vi "Dashboard Main.vi"() -> ()   [LabVIEW 2016]
uses:
  <vilib>/Utility/miscctls.llb/LVRowAndColumnTypeDef.ctl
  <vilib>/event_ctls.llb/eventvkey.ctl
  <vilib>/Rock Robotics/Network Tables/NT Read Numeric Array.vi
  <vilib>/Rock Robotics/Network Tables/NT Write Boolean.vi
  <vilib>/Rock Robotics/WPI/Dashboard/WPI_DashboardLogging Global.vi
panel:
  out "Background":bool
  in  "Camera Settings Right":T1={"Frame Rate"=30, "Compression"=30, "Size"=1, "DB Camera Config"=FALSE} {"Frame Rate" scale=1.0..30.0; "Compression" scale=100.0..-1.0; "Size" items=["640x480", "320x240", "160x120"]}
  in  "Camera Name Right":string(combo)="No Camera Selection"
  out "Camera Info":cluster{"Mbps LED":bool, "Mbps":dbl, "fps":dbl} {"fps" format="%#.1g"; "Mbps" format="%#.1g"}
  in  "Camera Settings":T1={"Frame Rate"=30, "Compression"=30, "Size"=1, "DB Camera Config"=FALSE} {"Frame Rate" scale=1.0..30.0; "Compression" scale=100.0..-1.0; "Size" items=["640x480", "320x240", "160x120"]}
  in  "TCP":refnum<k5>
  in  "Rec Mode":enum32{"Stop", "Record", "Playback"}(radio)
  out "Robot IP":string
  out "Image Message":string="Timeout in Camera Communications"
  in  "Dashboard Tab":T2(tab)
  in  "Smooth":i32(knob) scale=1.0..4.0
  in  "GoFast":bool
  in  "Select Auto":string(combo)="Select Autonomous ..."
  out "NT Connection":bool
  out "MotorChart R":cluster{"Numeric":dbl, "Numeric":dbl}(graph)
  out "MotorChart L":cluster{"Numeric":dbl, "Numeric":dbl}(graph)
  out "MotorSliders R":cluster{"MotorSlide1":dbl, "MotorSlide2":dbl} {"MotorSlide2" scale=-1.0..1.0 scale format="%#_2e"; "MotorSlide1" scale=-1.0..1.0 scale format="%#_2e"}
  out "MotorSliders L":cluster{"MotorSlide1":dbl, "MotorSlide2":dbl} {"MotorSlide2" scale=-1.0..1.0 scale format="%#_2e"; "MotorSlide1" scale=-1.0..1.0 scale format="%#_2e"}
  out "Gyro":dbl(knob) scale=0.0..360.0
  out "JS1 Z":dbl(slide) scale=-1.0..1.0 scale format="%#_2e"
  out "JS1 Graph":cluster{"X":dbl, "Y":dbl}[](graph)
  out "JS1 Buttons":T3
  out "JS2 Z":dbl(slide) scale=-1.0..1.0 scale format="%#_2e"
  out "JS2 Graph":cluster{"X":dbl, "Y":dbl}[](graph)
  out "JS2 Buttons":T3
  out "Mode":T4(ring)=enum."Auto Disabled"
  in  "Trim":dbl(slide)=0.5612244897959183 scale=0.0..1.0
  out "Sonar":dbl
  out "Camera Image Right":T5(plugin-control)
  in  "Calculate Angle":bool
  in  "Angle to turn":dbl=30.0
  out "Angle":dbl
  in  "Distance from\n lift to corner":dbl
  in  "Distance from \nthe lift to the wall":dbl
  in  "DB/String 4":string
  in  "DB/String 3":string
  in  "DB/String 2":string
  in  "DB/String 1":string
  in  "DB/String 0":string
  in  "DB/Slider 0":dbl(slide)=0.65 caption="Turning Speed" scale=0.0..1.0
  in  "DB/Slider 1":dbl(slide)=11.0 caption="Distance we stop\nfrom lift (in inches)" scale=0.0..30.0
  in  "DB/Slider 2":dbl(slide)=11.111111111111112 caption="Autonomous Stop" scale=0.0..50.0
  in  "DB/Slider 3":dbl(slide)=0.6565656565656566 caption="Autonomous Trim" scale=0.0..1.0
  out "DB/LED 3":bool
  out "DB/LED 2":bool
  out "DB/LED 1":bool
  out "DB/LED 0":bool
  in  "DB/Button 3":bool
  in  "DB/Button 2":bool
  in  "DB/Button 1":bool
  in  "DB/Button 0":bool caption="New Name"
  in  "Scaling factor (V/in)":dbl=0.0098
  out "distance":dbl(slide)=125.0 scale=0.0..250.0 scale format="%3d"
  out "Z Acceleration":dbl
  out "Y Acceleration":dbl
  out "X Acceleration":dbl
  in  "Test Slider":dbl(slide) scale=0.0..100.0 scale format="%#_3g"
  in  "On/Off":bool caption="Solenoid"
  in  "Test Name":u16(ring) items=["Select the test to run..."]
  in  "Test Tree":string(tree)
  in  "Motor":cluster{"Value":dbl, "Enable":bool} {"Value" scale=-1.0..1.0 scale format="%#_3g"}
  out "Progress":T6 {"Test Progress" scale=0.0..100.0}
  in  "Rev/Fwd":cluster{"Forward":bool, "Reverse":bool}
  in  "Test Ring":u16(ring) items=["Monochrome", "Color"]
  out "Cmd Status":string
  in  "Execute Command":bool
  in  "Command Params":string[][](table)
  in  "Command Selection":i32(listbox)
  in  "CheckList":i32(listbox)
  out "Tree":string(tree)
  out "Camera Image":T5(plugin-control)
  in  "Camera Name":string(combo)="No Camera Selection"
  # "HW"
  # "HW"
  # "Joysticks"
  # "Drive Motors"
  # "Front"
  # "Right"
  # "Left"
  # "Back"
  # "This tab is a great place for autonomous settings and robot-specific values.\nPlace controls and indicators inside this tab and match name to\nDashboard Variables on robot. You can also delete this comment."
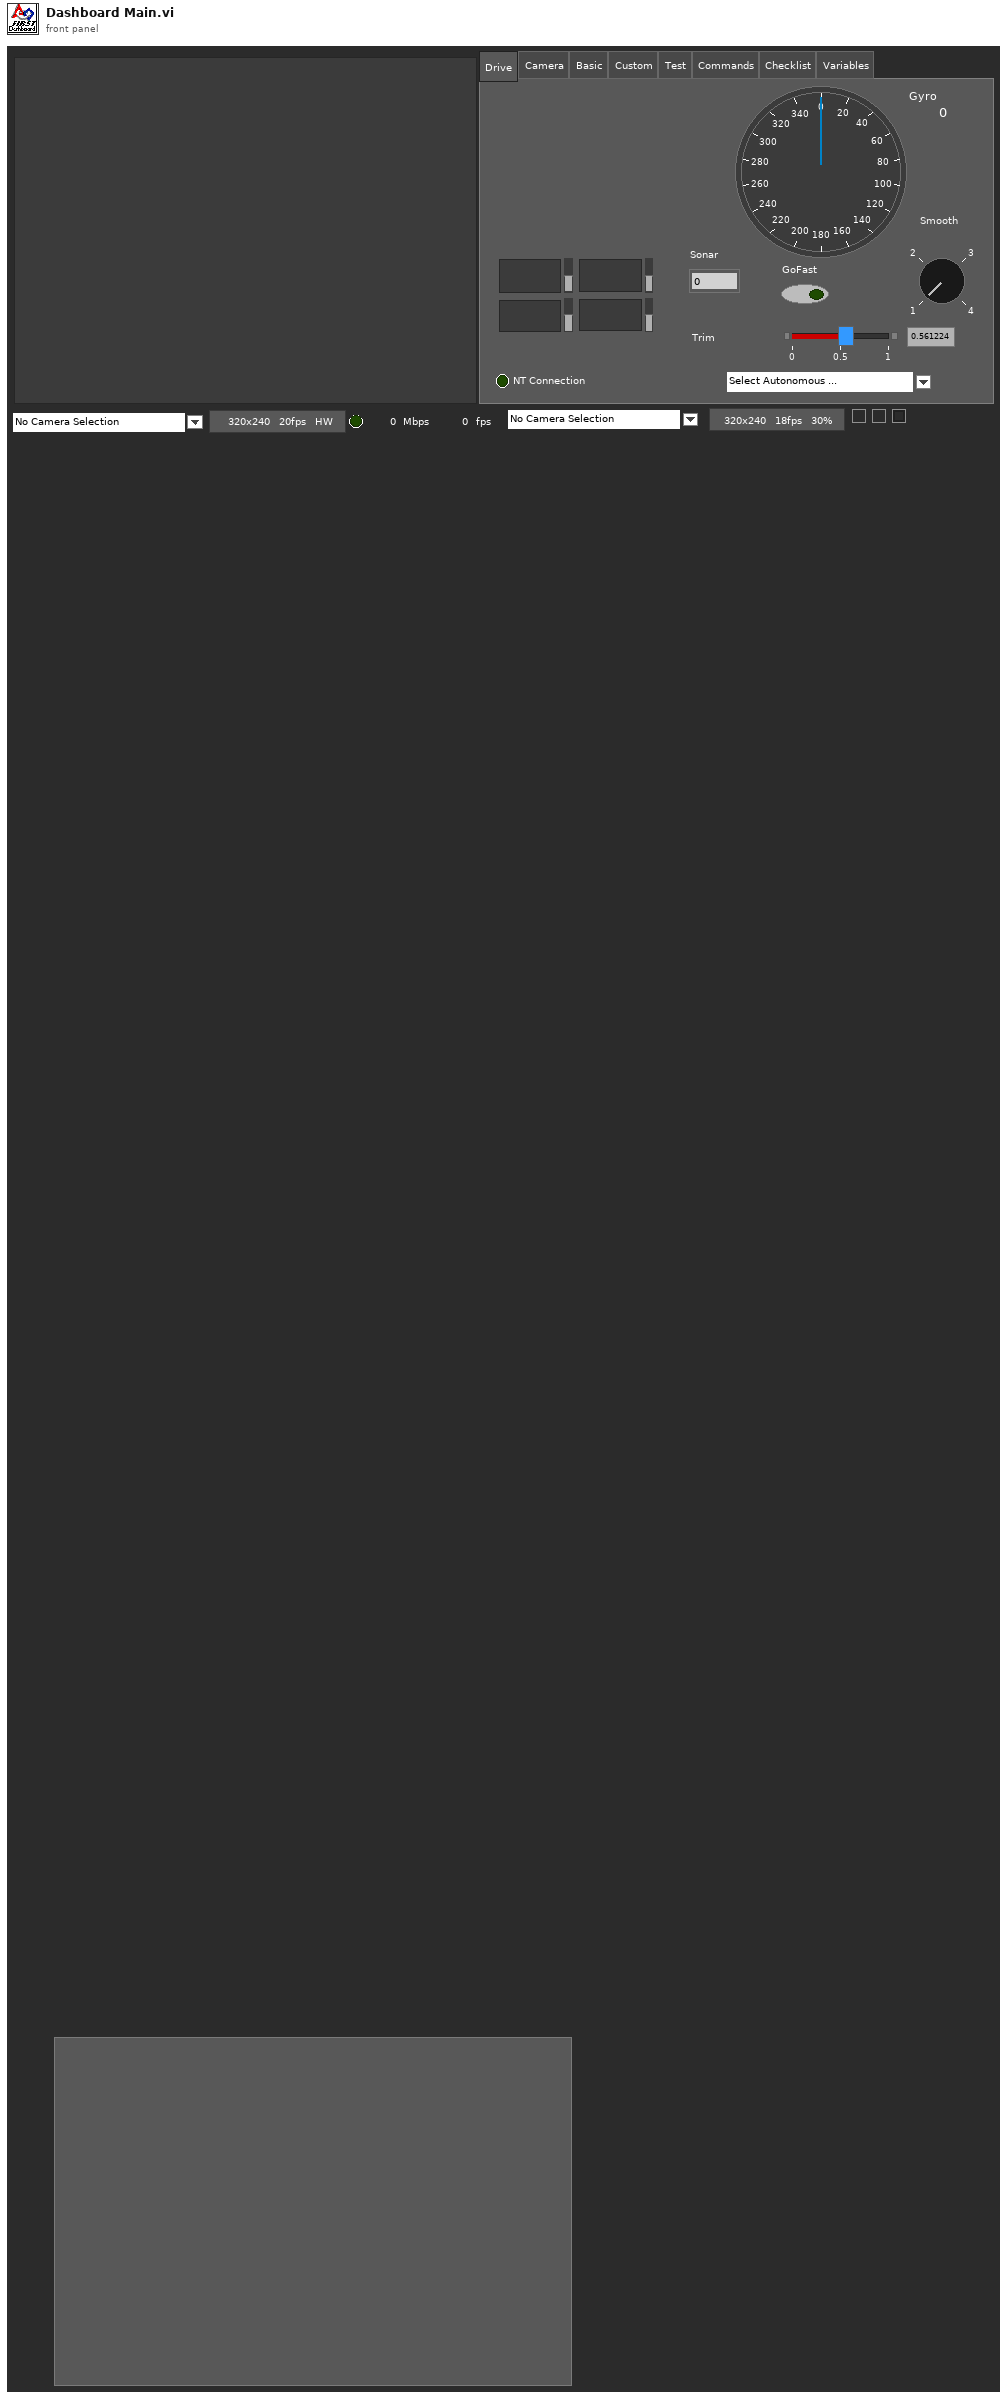
[diagram p1: front panel]
types:
  T1 = cluster{"Frame Rate":i32, "Compression":i32, "Size":u16, "DB Camera Config":bool}
  T2 = enum32{"Drive", "Camera", "Basic", "Custom", "Test", "Commands", "Checklist", "Variables"}
  T3 = cluster{bool, bool, bool, bool, bool, bool, bool, bool, bool, bool, bool, bool}
  T4 = enum8{"Tele-Op Disabled", "Tele-Op Enabled", "Auto Disabled", "Auto Enabled", "Test Disabled", "Test Enabled", "Disconnected", "No Code", "E-Stop"}
  T5 = typedef "IMAQ Image.ctl" = refnum<image>
  T6 = cluster{"Test Progress":u8, "Test Progress Text":string}
  T7 = typedef "Image Type" = u32
  T8 = cluster{"IDs":cluster{"RPC field ID":u16, "Unique ID":u16}, "String":string}
  T9 = enum32{"Drive", "Basic", "Custom", "Test", "Checklist", "Variables"}
  T10 = cluster{"Error Strings":string, "Disable Counts":cluster{u16, u16}, "Rail Faults":cluster{u16, u16, u16}, "Robot IP":string, "DB Mode":u8, "Event Info":cluster{"Name":string, "Type":u8, "Number":u16, "Replay":u8}}
  T11 = cluster{"Storage":cluster{"Disk Free":u64, "RAM Block":u32, "RAM free":u32}, "CPU Utilization":cluster{"CPU % ISR":sgl, "CPU % Time Crit":sgl, "CPU % Timed Str":sgl, "CPU % High":sgl, "CPU % Above":sgl, "CPU % Normal":sgl, "CPU % Low":sgl}, "CAN":cluster{"% Bus Utilization":sgl, "Bus Off Cnt":u32, "TX_FIFO Full Cnt":u32, "Receive Error Cnt":u8, "Transmit Error Cnt":u8}, "HID":cluster{"HID Outputs":u32, "Rumble Low":u16, "Rumble High":u16}[]}
  T12 = cluster{"Status bits":cluster{"Test Mode":bool, "Autonomous":bool, "Enabled":bool, "Code Start":bool, "Brownout":bool, "Reserved 2":bool, "Reserved 3":bool, "E-Stop":bool}, "Code Trace":cluster{"Disabled":bool, "TeleOp":bool, "Auto":bool, "Test":bool}, "Controller Type":enum16{"unknown", "cRIO", "roboRio"}, "Code?":enum16{"unknown", "noCode", "code"}, "Battery V":dbl}
  T13 = cluster{"Control Bits":cluster{"TestMode":bool, "Autonomous":bool, "Enabled":bool, "FMS Present":bool, bool, bool, bool, "E-Stop":bool}, "Team Station ":u8, "Countdown":sgl, "Joystick Values":cluster{"Axes":dbl[], "Buttons":bool[], "POVs":i16[]}[]}
  T14 = cluster{"Axes":dbl[], "Buttons":bool[], "POVs":i16[]}[]
  T15 = cluster{"Axes":dbl[], "Buttons":bool[], "POVs":i16[]}
  T16 = cluster{"Buttons[0]":bool, "Buttons[1]":bool, "Buttons[2]":bool, "Buttons[3]":bool, "Buttons[4]":bool, "Buttons[5]":bool, "Buttons[6]":bool, "Buttons[7]":bool, "Buttons[8]":bool, "Buttons[9]":bool, "Buttons[10]":bool, "Buttons[11]":bool}
  T17 = cluster{"Camera Image":refnum<vi>, "Dashboard Tab":refnum<vi>, "Background":refnum<vi>, "Rec Mode":refnum<vi>, "Test Slider":refnum<vi>, "On/Off ":refnum<vi>, "Test Ring":refnum<vi>, "Rev/Fwd":refnum<vi>, "Test Name":refnum<vi>, "Motor":refnum<vi>, "Progress":refnum<vi>, "CheckList":refnum<vi>, "Tree":refnum<vi>, "Test Tree":refnum<vi>, "Command Params":refnum<vi>, "Command Selection":refnum<vi>, "Execute Command":refnum<vi>, "Cmd Status":refnum<vi>, "Camera Settings":refnum<vi>, "Camera Name":refnum<vi>, "Camera Info":refnum<vi>, "Camera Settings Right":refnum<vi>, "Camera Name Right":refnum<vi>, "Camera Image Right":refnum<vi>}
  T18 = cluster{"Operation":enum16{"Update", "Clear"}, "Color Box":u32}[]
  T19 = typedef "eventvkey.ctl" = enum16{"ASCII", "Enter", "Return", "Shift", "Ctrl", "Alt", "Cmd", "Opt", "Caps", "NumLock", "Clear", "Break", "Up", "Down", "Left", "Right", "Insert", "Delete", "Home", "End", "PageUp", "PageDown", "Escape", "Help", "Pause", "ScrollLock", "F1", "F2", "F3", "F4", "F5", "F6", "F7", "F8", "F9", "F10", "F11", "F12", "F13", "F14", "F15", "F16", "F17", "F18", "F19", "F20", "F21", "F22", "F23", "F24", "Play", "VolumeUp", "VolumeDown", "Mute", "Two Byte Char"}
  T20 = cluster{"Image Size":bool, "Image Type":bool, "Pixel Value":bool, "ROI Information":bool, "Zoom Factor":bool}
  T21 = cluster{"Operation":enum16{"Update", "Clear"}, "Color Box":u32}
  T22 = typedef "LVRowAndColumnTypeDef.ctl" = cluster{"Row":i32, "Column":i32}
  T23 = cluster{"Shift":bool, "Ctrl":bool, "Alt":bool, "Cmd":bool, "Opt":bool}
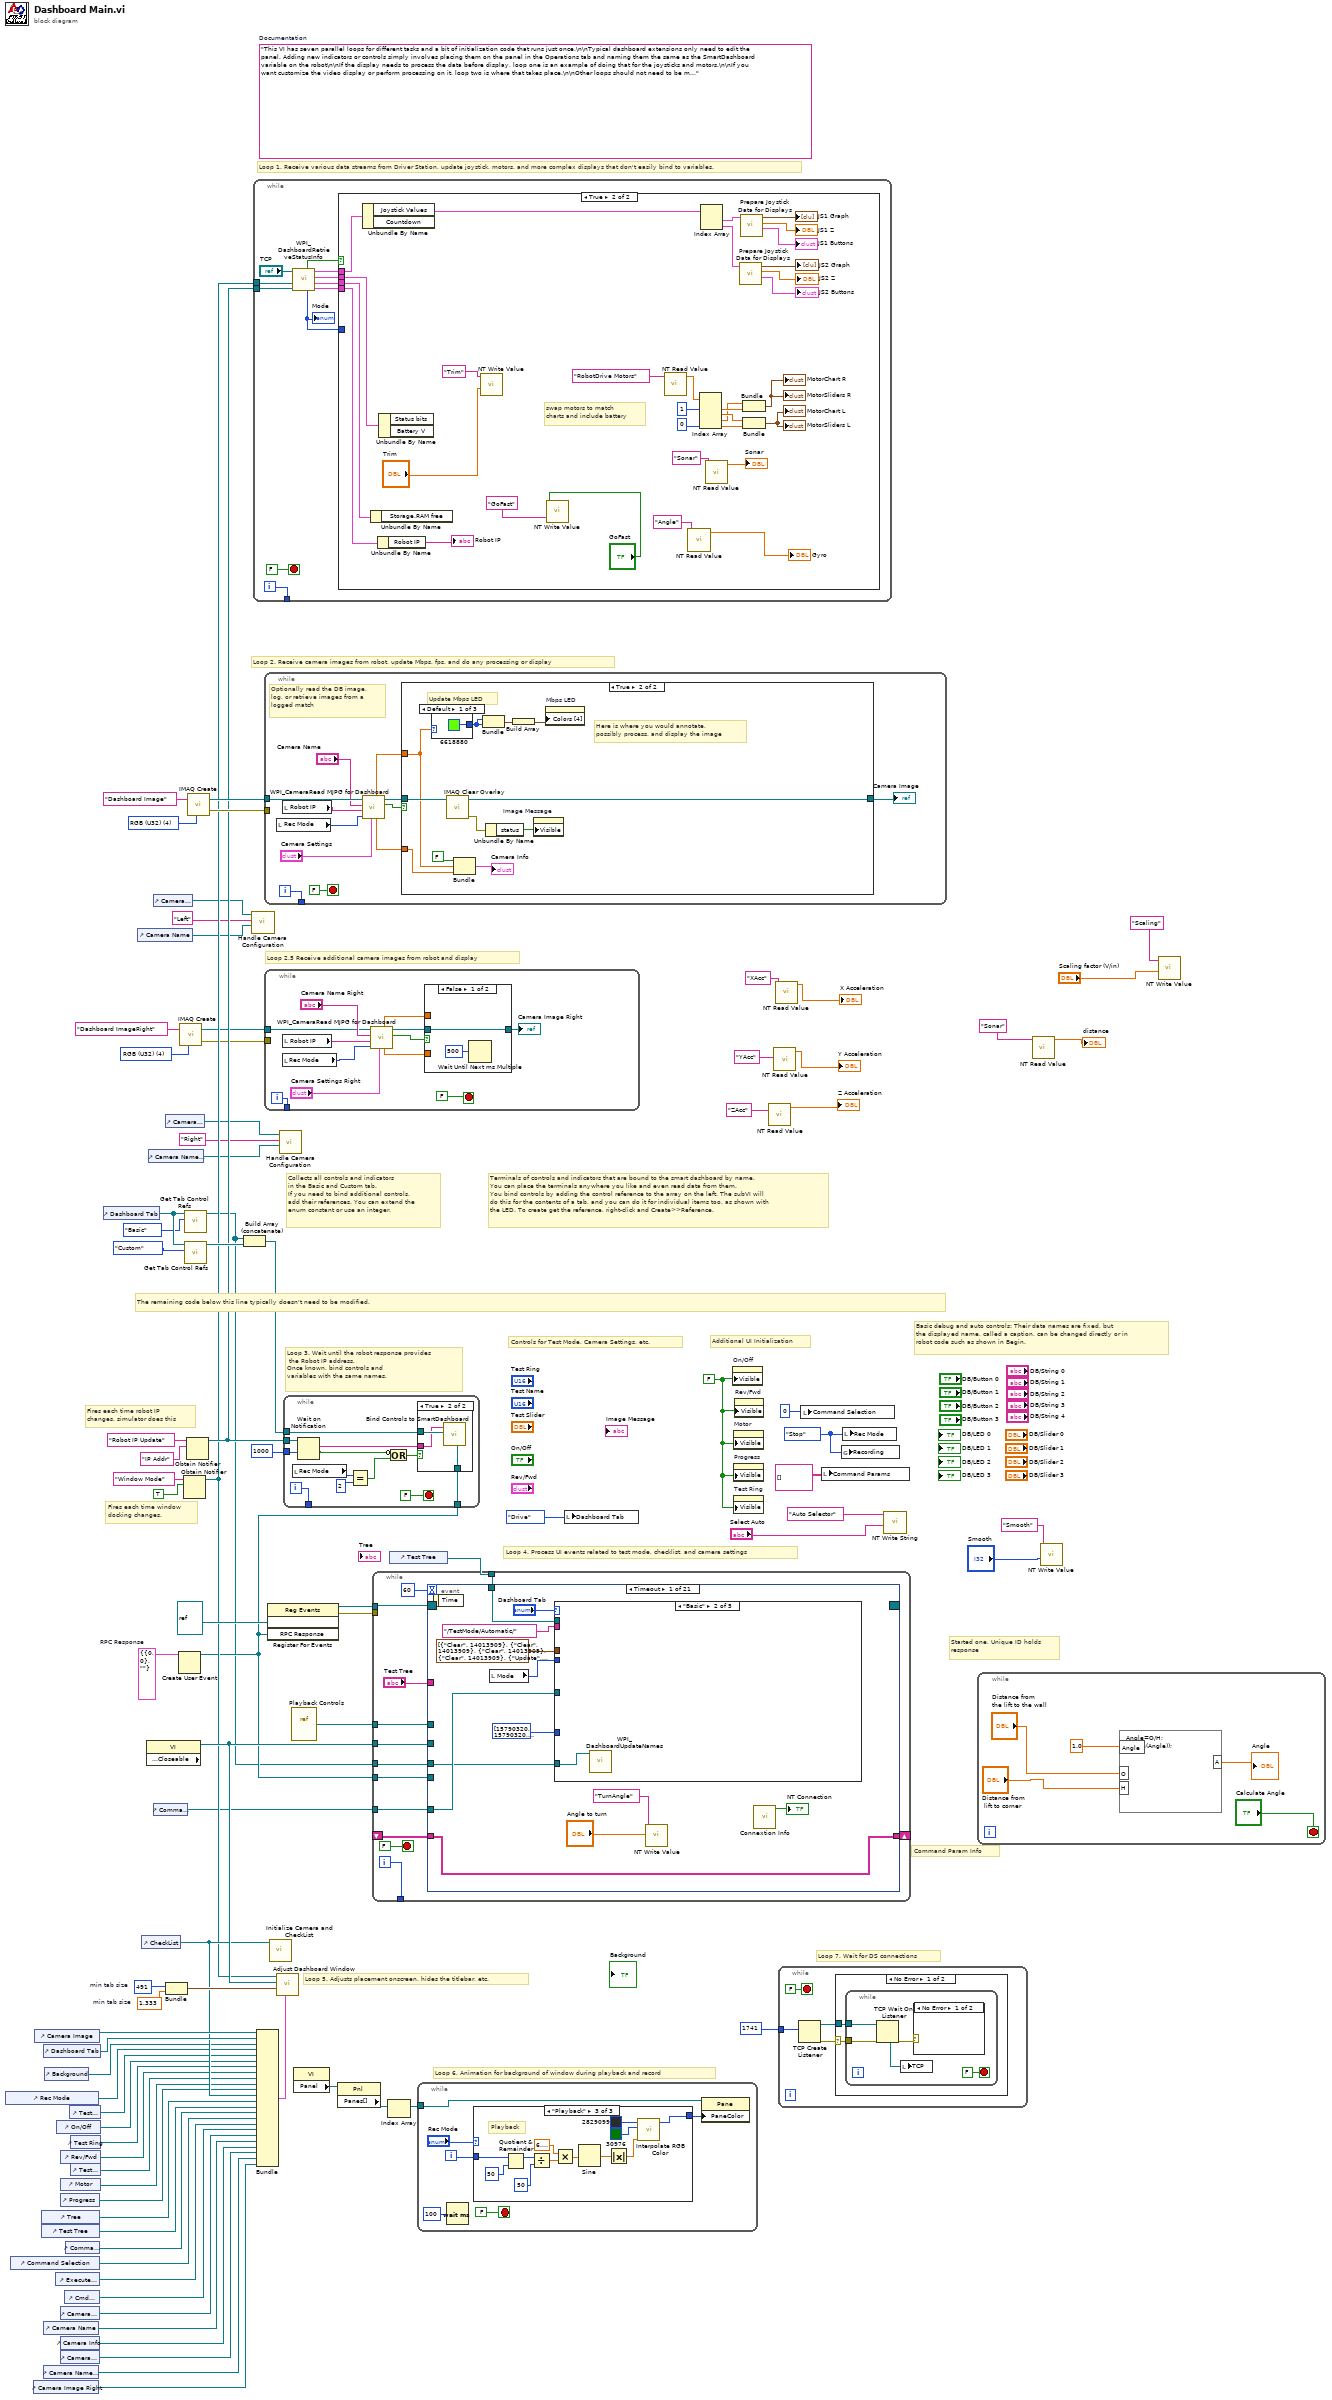
[diagram p0: block diagram]
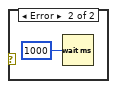
[diagram p3: hidden frame]
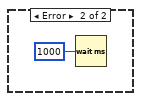
[diagram p4: hidden frame]
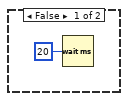
[diagram p5: hidden frame]
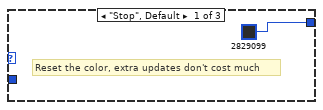
[diagram p6: hidden frame]
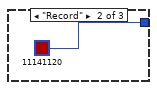
[diagram p7: hidden frame]
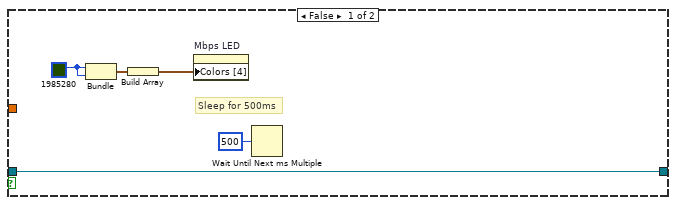
[diagram p9: hidden frame]
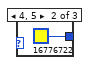
[diagram p10: hidden frame]
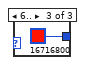
[diagram p11: hidden frame]
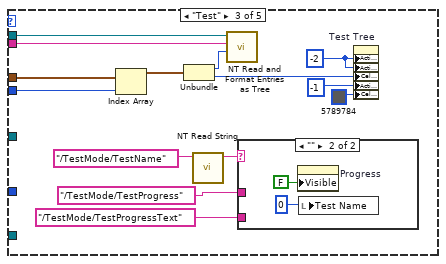
[diagram p13: hidden frame]
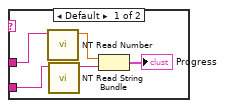
[diagram p14: hidden frame]
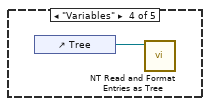
[diagram p15: hidden frame]
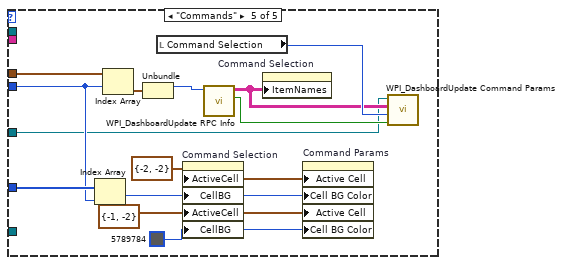
[diagram p16: hidden frame]
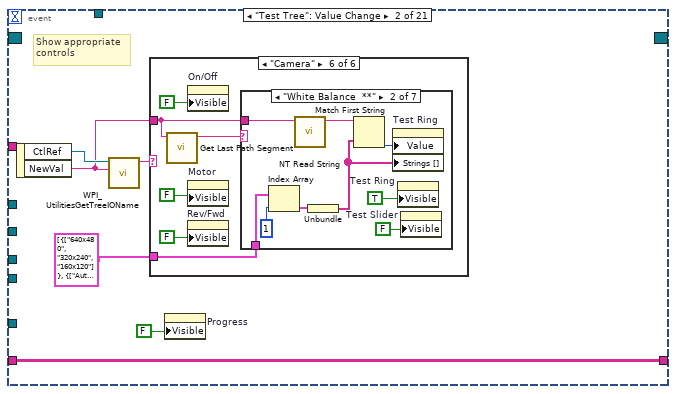
[diagram p17: hidden frame]
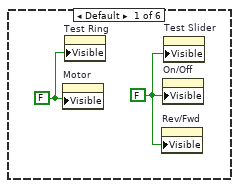
[diagram p18: hidden frame]
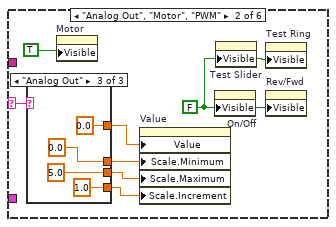
[diagram p19: hidden frame]
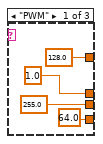
[diagram p20: hidden frame]
diagram:
  w24 = T7 4 items=["Grayscale (U8)", "Grayscale (I16)", "Grayscale (SGL)", "Complex (CSG)", "RGB (U32)", "HSL (U32)", "RGB (U64)"] ("Image Type")
  w40 = T8 {"IDs"={"RPC field ID"=0, "Unique ID"=0}, "String"=""}  # RPC Response
  w63 = 491  # min tab size
  w62 = 1.333  # min tab size
  w70 = enum32{"Stop", "Record", "Playback"}."Stop" ("Rec Mode")
  w47 = FALSE ("Visible")
  (unwired) "This VI has seven parallel loops for different tasks and a bit of initialization code that runs just once.\n\nTypical dashboard extensions only need to edit the panel. Adding new indicators or controls simply involves placing them on the panel in the Operations tab and naming them the same as the SmartDashboard variable on the robot\n\nIf the display needs to process the data before display, loop one is an example of doing that for the joysticks and motors.\n\nIf you want customize the video display or perform processing on it, loop two is where that takes place.\n\nOther loops should not need to be modified. They are pretty standard, and document the task they perform."  # Documentation
  w87 = T7 4 items=["Grayscale (U8)", "Grayscale (I16)", "Grayscale (SGL)", "Complex (CSG)", "RGB (U32)", "HSL (U32)", "RGB (U64)"] ("Image Type")
  # "Loop 2.5 Receive additional camera images from robot and display"
  # "Command Param Info"
  # "Started one, Unique ID holds\nresponse"
  # "Loop 7. Wait for DS connections"
  # "Basic debug and auto controls: Their data names are fixed, but\nthe displayed name, called a caption, can be changed directly or in\nrobot code such as shown in Begin."
  # "Controls for Test Mode, Camera Settings, etc."
  # "Additional UI Initialization"
  # "Loop 6. Animation for background of window during playback and record"
  # "Fires each time robot IP\nchanges, simulator does this"
  # "Fires each time window\ndocking changes."
  # "Collects all controls and indicators\nin the Basic and Custom tab.\nIf you need to bind additional controls,\nadd their references. You can extend the\nenum constant or use an integer."
  # "The remaining code below this line typically doesn't need to be modified."
  # "Loop 4. Process UI events related to test mode, checklist, and camera settings"
  # "Terminals of controls and indicators that are bound to the smart dashboard by name.\nYou can place the terminals anywhere you like and even read data from them.\nYou bind controls by adding the control reference to the array on the left. The subVI will\ndo this for the contents of a tab, and you can do it for individual items too, as shown with\nthe LED. To create get the reference, right-click and Create>>Reference."
  # "Loop 3. Wait until the robot response provides\n the Robot IP address.\nOnce known, bind controls and\nvariables with the same names."
  # "Loop 5. Adjusts placement onscreen, hides the titlebar, etc."
  # "Loop 1. Receive various data streams from Driver Station, update joystick, motors, and more complex displays that don't easily bind to variables."
  # "Loop 2. Receive camera images from robot, update Mbps, fps, and do any processing or display"
  n1 = control-ref of="Rec Mode"() -> (w53:refnum<vi>)
  n2 = control-ref of="Command Selection"() -> (w39:refnum<vi>)
  n3 = control-ref of="Camera Image Right"() -> (w15:refnum<vi>)
  n4 = control-ref of="Camera Image"() -> (w65:refnum<vi>)
  n5 = control-ref of="Tree"() -> (w57:refnum<vi>)
  n6 = control-ref of="Test Tree"() -> (w56:refnum<vi>)
  n7 = control-ref of="Dashboard Tab"() -> (w64:refnum<vi>)
  n8 = control-ref of="Camera Name"() -> (w30:refnum<vi>)
  n9 = control-ref of="Camera Name Right"() -> (w16:refnum<vi>)
  n10 = control-ref of="Background"() -> (w13:refnum<vi>)
  n11 = control-ref of="Execute Command"() -> (w41:refnum<vi>)
  n12 = control-ref of="On/Off"() -> (w51:refnum<vi>)
  n13 = control-ref of="Progress"() -> (w48:refnum<vi>)
  n14 = control-ref of="Camera Settings"() -> (w31:refnum<vi>)
  n15 = control-ref of="Camera Info"() -> (w29:refnum<vi>)
  n16 = control-ref of="Camera Settings Right"() -> (w17:refnum<vi>)
  n17 = control-ref of="Rev/Fwd"() -> (w49:refnum<vi>)
  n18 = control-ref of="Motor"() -> (w54:refnum<vi>)
  n19 = control-ref of="Cmd Status"() -> (w35:refnum<vi>)
  n20 = control-ref of="Command Params"() -> (w42:refnum<vi>)
  n21 = control-ref of="Test Slider"() -> (w52:refnum<vi>)
  n22 = control-ref of="Test Ring"() -> (w50:refnum<vi>)
  n23 = control-ref of="Test Name"() -> (w55:refnum<vi>)
  n24 = control-ref of="Dashboard Tab"() -> (w68:refnum<vi>)
  n25 = control-ref of="Camera Name"() -> (w32:refnum<vi>)
  n26 = control-ref of="CheckList"() -> (w58:refnum<vi>)
  n27 = property class="VI" props=["Front Panel.Closeable"]() -> (reference out=w69:refnum<vi>)  [unwired: 2 in, 2 out]
  n28 = control-ref of="Camera Name Right"() -> (w20:refnum<vi>)
  n29 = control-ref of="Camera Settings"() -> (w33:refnum<vi>)
  n30 = control-ref of="Command Params"() -> (w34:refnum<vi>)
  n31 = control-ref of="Camera Settings Right"() -> (w21:refnum<vi>)
  n32 = Bundle("min tab size"=w63, "min tab size"=w62) -> (w61:cluster{"min tab size":i32, "min tab size":dbl})  [unwired: 1 in]
  n33 = Create User Event(user event datatype=w40) -> (user event=w36:refnum<user-event>)  [unwired: 1 in, 1 out]
  n34 = call "IMAQ Create"("Image Name"="Dashboard ImageRight", "Image Type"=w24) -> ("New Image"=w23:T5, "error out"=w22:errorcluster)  [unwired: 2 in, 1 out]
  n35 = Obtain Notifier(name (unnamed)="Window Mode", notification data type=TRUE) -> (notifier out=w45:refnum<notifier>)  [unwired: 2 in, 2 out]
  n36 = call <vilib>:"Get Tab Control Refs.vi"("Page Index"=T9."Basic" ("Dashboard Tab"), "TabControl in"=w68) -> ("ControlsOnPage"=w28:refnum<vi>[])  [unwired: 9 in]
  n37 = call <vilib>:"Get Tab Control Refs.vi"("Page Index"=T9."Custom" ("Dashboard Tab"), "TabControl in"=w68) -> ("ControlsOnPage"=w67:refnum<vi>[])  [unwired: 9 in]
  n38 = Obtain Notifier(name (unnamed)="Robot IP Update", notification data type="IP Addr" ("name (unnamed)")) -> (notifier out=w46:refnum<notifier>)  [unwired: 2 in, 2 out]
  n39 = call "IMAQ Create"("Image Name"="Dashboard Image", "Image Type"=w87) -> ("New Image"=w85:T5, "error out"=w84:errorcluster)  [unwired: 2 in, 1 out]
  n40 = Build Array (concatenate)(w28, w67) -> (w66:refnum<vi>[])
  n41 = call "Handle Camera Configuration.vi"("CameraNameRef"=w32, "Camera File Name"="Left", "ClusterRef"=w33) -> ()  [unwired: 9 in]
  n42 = while {
    tunnel: [w97] -> _
    tunnel: w46 -> [w91]
    tunnel: w45 -> [w88]
    i -> [w97]
    stop <- FALSE stop-if-true
    n43 = call <vilib>:"WPI_DashboardRetrieveStatusInfo.vi"("Binding Refnum"=w91, "Window Mode Notifier"=w88, "TCP Cnx"="TCP") -> ("Power and Errors"=w92:T10, "Robot Metrics"=w95:T11, "Status Info"=w96:T12, "Control Info"=w93:T13, "Robot Mode"=w90:T4, "Process?"=w94:bool)  [unwired: 3 in]
    "Mode" <- w90
    n44 = case shown="True" w94 {
      tunnel: w96 -> [_ w131]
      tunnel: w95 -> [_ w130]
      tunnel: w93 -> [_ w129]
      tunnel: w92 -> [_ w128]
      tunnel: w90 -> [_ _]
      frame False {
        n45 = Wait (ms)(milliseconds to wait=u32 20) -> ()  [unwired: 1 out]
      }
      frame True {
        # "swap motors to match\ncharts and include battery"
        n46 = Unbundle By Name(w129) -> ("Joystick Values"=w119:T14)  [unwired: 1 out]
        n47 = Unbundle By Name(w130) -> ()  [unwired: 1 out]
        n48 = Unbundle By Name(w128) -> ("Robot IP"=→"Robot IP":string)
        n49 = Unbundle By Name(w131) -> ()  [unwired: 2 out]
        n50 = call-poly <vilib>:"NT Write Value.vi"("Numeric"="Trim", "Name"="Trim") -> ()  [unwired: 9 in, 1 out]
        n51 = call-poly <vilib>:"NT Write Value.vi"("Boolean"="GoFast", "Name"="GoFast") -> ()  [unwired: 9 in, 1 out]
        n52 = call-poly <vilib>:"NT Read Value.vi"("Name"="RobotDrive Motors") -> ("Numeric Array"=w109:dbl[])  [unwired: 9 in, 1 out]
        n53 = call-poly <vilib>:"NT Read Value.vi"("Name"="Angle") -> ("Numeric"=→"Gyro":dbl)  [unwired: 9 in, 1 out]
        n54 = Index Array(array=w109, index #1=1, index #4=0) -> (element #1=w123:dbl, element #2=w124:dbl, element #3=w122:dbl, element #4=w127:dbl)  [unwired: 2 in]
        n55 = Index Array(array=w119) -> (element #1=w118:T15, element #2=w114:T15)  [unwired: 2 in]
        n56 = call-poly <vilib>:"NT Read Value.vi"("Name"="Sonar") -> ("Numeric"=→"Sonar":dbl)  [unwired: 9 in, 1 out]
        n57 = call "Prepare Joystick Data for Displays.vi"("Joystick Values"=w114) -> ("Buttons"=→"JS2 Buttons":T16, "Z Axis"=→"JS2 Z":dbl, "Cartesian Data"=→"JS2 Graph":cluster{"X axis":dbl, "X axis":dbl}[])  [unwired: 8 in]
        n58 = call "Prepare Joystick Data for Displays.vi"("Joystick Values"=w118) -> ("Buttons"=→"JS1 Buttons":T16, "Z Axis"=→"JS1 Z":dbl, "Cartesian Data"=→"JS1 Graph":cluster{"X axis":dbl, "X axis":dbl}[])  [unwired: 8 in]
        n59 = Bundle("Numeric"=w122, "Numeric"=w123) -> (→"MotorChart R" →"MotorSliders R":cluster{"Numeric":dbl, "Numeric":dbl})  [unwired: 1 in]
        n60 = Bundle("Numeric"=w124, "Numeric"=w127) -> (→"MotorChart L" →"MotorSliders L":cluster{"Numeric":dbl, "Numeric":dbl})  [unwired: 1 in]
      }
    }
  }
  n61 = Bundle("Camera Image"=w65, "Dashboard Tab"=w64, "Background"=w13, "Rec Mode"=w53, "Test Slider"=w52, "On/Off"=w51, "Test Ring"=w50, "Rev/Fwd"=w49, "Test Name"=w55, "Motor"=w54, "Progress"=w48, "CheckList"=w58, "Tree"=w57, "Test Tree"=w56, "Command Params"=w42, "Command Selection"=w39, "Execute Command"=w41, "Cmd Status"=w35, "Camera Settings"=w31, "Camera Name"=w30, "Camera Info"=w29, "Camera Settings Right"=w17, "Camera Name Right"=w16, "Camera Image Right"=w15) -> (w14:T17)  [unwired: 1 in]
  n62 = while {
    tunnel: w85 -> [w141]
    tunnel: w84 -> [_]
    tunnel: [w142] -> _
    i -> [w142]
    stop <- FALSE stop-if-true
    # "Optionally read the DB image,\nlog, or retrieve images from a\nlogged match"
    n63 = local read "Rec Mode"() -> (w137:enum32{"Stop", "Record", "Playback"})
    n64 = local read "Robot IP"() -> (w136:string)
    n65 = call <vilib>:"WPI_CameraRead MJPG for Dashboard.vi"("Camera Settings"="Camera Settings", "Rec Mode"=w137, "Robot IP"=w136, "Camera Name"="Camera Name", "Refnum in"=w141) -> ("Active"=w139:bool, "Refnum out"=w140:T5, "FPS"=w138:dbl, "Bandwidth (Mbps)"=w135:dbl)  [unwired: 3 in]
    n66 = case shown="True" w139 {
      tunnel: w140 -> [w144 w155]
      tunnel: w135 -> [_ w152]
      tunnel: w138 -> [_ w153]
      tunnel: [w144 w149] -> w132
      frame False {
        w146 = u32 1985280 ("Color Box")
        # "Sleep for 500ms"
        n67 = Bundle("Color Box"=w146, "Color Box"=w146) -> (w147:cluster{"Color Box":u32, "Color Box":u32})  [unwired: 1 out]
        n68 = Build Array(w147) -> (w145:cluster{"Color Box":u32, "Color Box":u32}[])
        n69 = property on="Mbps LED" class="Bool (strict)"("Colors [4]"=w145) -> ()  [unwired: 2 in, 2 out]
        n70 = Wait Until Next ms Multiple(millisecond multiple=u32 500) -> ()  [unwired: 1 out]
      }
      frame True {
        # "Here is where you would annotate,\npossibly process, and display the image"
        # "Update Mbps LED"
        n71 = case shown="Default" w152 {
          tunnel: [u32 6618880 ("Color Box") u32 16776722 ("Color Box") u32 16716800 ("Color Box")] -> w156
          frame Default {
          }
          frame 4, 5 {
          }
          frame 6.. {
          }
        }
        n72 = call "IMAQ Clear Overlay"("Image"=w155) -> ("error out"=w158:errorcluster, "Image Out"=w149:T5)  [unwired: 2 in, 7 out]
        n73 = Bundle(FALSE, "Bandwidth (Mbps)"=w152, "FPS"=w153) -> (→"Camera Info":cluster{bool, "Bandwidth (Mbps)":dbl, "FPS":dbl})  [unwired: 1 in]
        n74 = Bundle("Color Box"=w156, "Color Box"=w156) -> (w157:cluster{"Color Box":u32, "Color Box":u32})  [unwired: 1 out]
        n75 = Unbundle By Name(w158) -> ("status"=w159:bool)
        n76 = Build Array(w157) -> (w154:cluster{"Color Box":u32, "Color Box":u32}[])
        n77 = property on="Image Message" class="Str"("Visible"=w159) -> ()  [unwired: 2 in, 2 out]
        n78 = property on="Mbps LED" class="Bool (strict)"("Colors [4]"=w154) -> ()  [unwired: 2 in, 2 out]
      }
    }
    "Camera Image" <- w132
  }
  n79 = while {
    tunnel: w23 -> [w173]
    tunnel: w22 -> [_]
    tunnel: [w167] -> _
    i -> [w167]
    stop <- FALSE stop-if-true
    n80 = local read "Rec Mode"() -> (w171:enum32{"Stop", "Record", "Playback"})
    n81 = local read "Robot IP"() -> (w172:string)
    n82 = call <vilib>:"WPI_CameraRead MJPG for Dashboard.vi"("Camera Settings"="Camera Settings Right", "Rec Mode"=w171, "Robot IP"=w172, "Camera Name"="Camera Name Right", "Refnum in"=w173) -> ("Active"=w166:bool, "Refnum out"=w169:T5, "FPS"=w164:dbl, "Bandwidth (Mbps)"=w165:dbl)  [unwired: 3 in]
    n83 = case shown="False" w166 {
      tunnel: w169 -> [w175 w177]
      tunnel: w165 -> [_ _]
      tunnel: w164 -> [_ _]
      tunnel: [w175 w177] -> w163
      frame False {
        n84 = Wait Until Next ms Multiple(millisecond multiple=u32 500) -> ()  [unwired: 1 out]
      }
      frame True {
      }
    }
    "Camera Image Right" <- w163
  }
  n85 = register-events(refnum<vi> refnum, w36) -> (reference out=w74:refnum<event-registration>, error out=w73:errorcluster)  [unwired: 2 in]
  n86 = call "Initialize Camera and CheckList.vi"("ListBox in"=w58) -> ()  [unwired: 11 in]
  n87 = call "Adjust Dashboard Window.vi"("Sizing Refnums"=w14, "Size Constraints"=w61, "VI"=w69, "WIn Mode"=w45) -> ()  [unwired: 8 in]
  n88 = call "Handle Camera Configuration.vi"("CameraNameRef"=w20, "Camera File Name"="Right", "ClusterRef"=w21) -> ()  [unwired: 9 in]
  n89 = while {
    tunnel: w66 -> [w189]
    tunnel: w46 -> [w187]
    tunnel: [w185] -> _
    tunnel: u32 1000 ("milliseconds to wait") -> [w184]
    tunnel: w36 -> [w178]
    i -> [w185]
    stop <- FALSE stop-if-true
    n90 = local read "Rec Mode"() -> (w180:enum32{"Stop", "Record", "Playback"})
    n91 = Wait on Notification(notifier=w187, timeout in ms (-1)=w184) -> (notification=w186:string, timed out?=w182:bool)  [unwired: 2 in, 2 out]
    n92 = Equal?(x=w180, y=u16 2 ("Rec Mode")) -> (x = y?=w181:bool)
    n93 = Compound Arithmetic op=OR(invert w182, w181) -> (w183:bool)
    n94 = case shown="True" w183 {
      tunnel: w189 -> [_ w192]
      tunnel: w186 -> [_ w191]
      tunnel: w178 -> [_ w190]
      frame False {
      }
      frame True {
        n95 = call <vilib>:"Bind Controls to SmartDashboard.vi"("RPC ref"=w190, "Bound Control Refs"=w192, "Server IP Address"=w191) -> ()  [unwired: 9 in]
      }
    }
  }
  n96 = vi-ref "Playback Controls.vi"() -> (w75:refnum<vi>)
  n97 = property class="VI"() -> ("Panel"=w77:refnum<vi>)  [unwired: 2 in, 2 out]
  n98 = property class="Pnl"(reference=w77) -> ("Panes[]"=w78:refnum<vi>[])  [unwired: 1 in, 2 out]
  n99 = Index Array(array=w78) -> (element=w76:refnum<vi>)  [unwired: 1 in]
  n100 = control-ref of="Test Tree"() -> (w79:refnum<vi>)
  n101 = while {
    tunnel: [w202] -> _
    tunnel: w79 -> [w201]
    tunnel: w75 -> [w200]
    tunnel: w74 -> [w199]
    tunnel: w73 -> [_]
    tunnel: w69 -> [w198]
    tunnel: w36 -> [w197]
    tunnel: w34 -> [w196]
    shift-right: [w195] -> _
    shift-left: _ -> [w194]
    tunnel: w28 -> [w193]
    i -> [w202]
    stop <- FALSE stop-if-true
    n102 = event shown="[0] Timeout" {
      selector: w199 -> [_ _ _ _ _ _ _ _ _ _ _ _ _ _ _ _ _ _ _ _ _]
      dyn-events: [_ _ _ _ _ _ _ _ _ _ _ _ _ _ _ _ w460 _ _ _ _] -> _
      timeout: u32 60 ("milliseconds to wait") -> [_ _ _ _ _ _ _ _ _ _ _ _ _ _ _ _ _ _ _ _ _]
      tunnel: w201 -> [w216 _ _ _ _ _ _ _ _ _ _ _ _ _ _ _ _ _ _ _ _]
      tunnel: "Test Tree" -> [_ _ _ _ _ _ _ _ _ _ _ w427 w435 w437 w441 w449 _ _ _ _ _]
      tunnel: w200 -> [_ _ _ _ _ _ _ _ _ _ _ _ _ _ _ _ w462 _ w480 _ _]
      tunnel: w198 -> [_ _ _ _ _ _ _ _ _ _ _ _ _ _ _ _ w458 _ _ _ _]
      tunnel: w197 -> [_ _ _ _ _ _ _ _ _ _ _ _ _ _ _ _ w454 _ _ _ _]
      tunnel: w196 -> [w211 _ _ _ _ _ w378 _ _ _ _ _ _ _ _ _ _ _ _ _ _]
      tunnel: [w210 w255 w357 w362 w371 w375 w376 w385 w395 w402 w414 w426 w433 w436 w440 w448 w453 w475 w477 w481 w492] -> w195
      tunnel: w194 -> [w210 w255 w357 w362 w371 w375 w376 _ _ w402 w414 w426 w433 w436 w440 w448 w453 w475 w477 w481 w492]
      tunnel: w193 -> [w208 _ _ _ _ _ _ _ _ _ _ _ _ _ _ _ _ _ _ _ _]
      event Timeout {
        n103 = event-data() -> ()  [unwired: 1 in, 1 out]
        n104 = local read "Mode"() -> (w213:T4)
        n105 = case shown="\"Basic\"" "Dashboard Tab" {
          tunnel: w216 -> [_ _ w232 _ _]
          tunnel: "/TestMode/Automatic/" ("Name Pattern") -> [_ _ w231 _ _]
          tunnel: T18 [{"Operation"=enum."Clear", "Color Box"=14013909}, {"Operation"=enum."Clear", "Color Box"=14013909}, {"Operation"=enum."Clear", "Color Box"=14013909}, {"Operation"=enum."Clear", "Color Box"=14013909}, {"Operation"=enum."Update", "Color Box"=14013909}, {"Operation"=enum."Update", "Color Box"=16777215}, {"Operation"=enum."Clear", "Color Box"=14013909}, {"Operation"=enum."Clear", "Color Box"=14013909}, {"Operation"=enum."Clear", "Color Box"=14013909}] -> [_ _ w224 _ w248]
          tunnel: w213 -> [_ _ w223 _ w247]
          tunnel: u32[] [15790320, 15790320, 15790320, 15790320, 16777215, 16777215, 15790320, 15790320, 15790320] -> [_ _ _ _ w253]
          tunnel: w211 -> [_ _ _ _ w241]
          tunnel: w208 -> [_ w218 _ _ _]
          frame "Custom", Default {
          }
          frame "Basic" {
            n106 = call <vilib>:"WPI_DashboardUpdateNames.vi"("Controls on Tab"=w218) -> ()  [unwired: 11 in]
          }
          frame "Test" {
            w230 = -2 ("Active Item:Row Number")
            n107 = Index Array(array=w224, index=w223) -> (element=w225:T21)
            n108 = Unbundle(w225) -> ("Operation"=w226:enum16{"Update", "Clear"}, "Color Box"=w227:u32)
            n109 = call <vilib>:"NT Read String.vi"("Name"="/TestMode/TestName") -> ("String"=w221:string)  [unwired: 9 in, 1 out]
            n110 = call <vilib>:"NT Read and Format Entries as Tree.vi"("Operation"=w226, "Name Pattern"=w231, "Tree Refnum"=w232) -> ()  [unwired: 7 in, 2 out]
            n111 = case shown="\"\"" w221 {
              tunnel: "/TestMode/TestProgress" ("Name") -> [w234 _]
              tunnel: "/TestMode/TestProgressText" ("Name") -> [w233 _]
              frame Default {
                n112 = call <vilib>:"NT Read Number.vi"("Name"=w234) -> ("Numeric"=w235:dbl)  [unwired: 9 in, 1 out]
                n113 = call <vilib>:"NT Read String.vi"("Name"=w233) -> ("String"=w236:string)  [unwired: 9 in, 1 out]
                n114 = Bundle("Numeric"=w235, "String"=w236) -> (→"Progress":cluster{"Numeric":dbl, "String":string})  [unwired: 1 in]
              }
              frame "" {
                n115 = property on="Progress" class="Clust (strict)"("Visible"=FALSE) -> ()  [unwired: 2 in, 2 out]
                n116 = local write "Test Name"(u16 0) -> ()
              }
            }
            n117 = property on="Test Tree" class="Tree (strict)"("Active Item Row Number"=w230, "ActiveColNum"=w230, "CellBG"=w227, "Active Item Row Number"=-1 ("Active Item:Row Number"), "CellBG"=u32 5789784 ("Color Box")) -> ()  [unwired: 2 in, 2 out]
          }
          frame "Variables" {
            n118 = control-ref of="Tree"() -> (w240:refnum<vi>)
            n119 = call <vilib>:"NT Read and Format Entries as Tree.vi"("Tree Refnum"=w240) -> ()  [unwired: 9 in, 2 out]
          }
          frame "Commands" {
            w249 = u32 5789784 ("Color Box")
            w250 = T22 {"Row"=-1, "Column"=-2} ("Active Cell:Active Cell")
            w252 = T22 {"Row"=-2, "Column"=-2} ("Active Cell:Active Cell")
            n120 = Index Array(array=w253, index=w247) -> (element=w251:u32)
            n121 = Index Array(array=w248, index=w247) -> (element=w246:T21)
            n122 = Unbundle(w246) -> ("Operation"=w245:enum16{"Update", "Clear"})  [unwired: 1 out]
            n123 = local read "Command Selection"() -> (w244:i32)
            n124 = property on="Command Selection" class="MCListbox (strict)"("ActiveCell"=w252, "CellBG"=w251, "ActiveCell"=w250, "CellBG"=w249) -> ()  [unwired: 2 in, 2 out]
            n125 = call <vilib>:"WPI_DashboardUpdate RPC Info.vi"("Operation"=w245) -> ("update"=w243:bool, "commands"=w242:string[][])  [unwired: 9 in]
            n126 = property on="Command Selection" class="MCListbox (strict)"("ItemNames"=w242) -> ()  [unwired: 2 in, 2 out]
            n127 = property on="Command Params" class="Tbl (strict)"("Active Cell"=w252, "Cell BG Color"=w251, "Active Cell"=w250, "Cell BG Color"=w249) -> ()  [unwired: 2 in, 2 out]
            n128 = call <vilib>:"WPI_DashboardUpdate Command Params.vi"("Update"=w243, "NewVal"=w244, "Commands"=w242, "Param Tbl"=w241) -> ()  [unwired: 7 in, 1 out]
          }
        }
        n129 = call-poly <vilib>:"NT Write Value.vi"("Numeric"="Angle to turn", "Name"="TurnAngle") -> ()  [unwired: 9 in, 1 out]
        n130 = call <vilib>:"Connextion Info.vi"() -> ("Connected"=→"NT Connection":bool)  [unwired: 10 in, 1 out]
      }
      event "Test Tree": Value Change {
        # "Show appropriate\ncontrols"
        n131 = event-data() -> ("CtlRef"=w258:refnum<vi>, "NewVal"=w256:string)  [unwired: 1 in]
        n132 = call <vilib>:"WPI_UtilitiesGetTreeIOName.vi"("NewVal"=w256, "TreeControl in"=w258) -> ("I/O Name"=w259:string)  [unwired: 9 in]
        n133 = case shown="\"Camera\"" w259 {
          selector: w259 -> [_ w266 _ w288 w297 _]
          tunnel: w256 -> [_ _ w285 w287 _ w304]
          tunnel: cluster{string[]}[] [{["640x480", "320x240", "160x120"]}, {["Auto", "Fixed indoor", "Fixed outdoor 1", "Fixed outdoor 2", "Fixed fluorescent 1", "Fixed fluorescent 2", "Hold current"]}, {["Auto", "Flicker-free 50 Hz", "Flicker-free 60 Hz", "Hold current"]}, {["None", "Prioritize frame rate", "Prioritize image quality"]}, {["Monochrome", "Color"]}] -> [_ _ _ _ _ w303]
          frame Default {
            w261 = FALSE ("Visible")
            w260 = FALSE ("Visible")
            n134 = property on="Motor" class="Clust (strict)"("Visible"=w260) -> ()  [unwired: 2 in, 2 out]
            n135 = property on="Test Ring" class="Ring (strict)"("Visible"=w260) -> ()  [unwired: 2 in, 2 out]
            n136 = property on="Rev/Fwd" class="Clust (strict)"("Visible"=w261) -> ()  [unwired: 2 in, 2 out]
            n137 = property on="On/Off" class="Bool (strict)"("Visible"=w261) -> ()  [unwired: 2 in, 2 out]
            n138 = property on="Test Slider" class="Slide (strict)"("Visible"=w261) -> ()  [unwired: 2 in, 2 out]
          }
          frame "Analog Out", "Motor", "PWM" {
            w267 = FALSE ("Visible")
            n139 = case shown="\"Analog Out\"" w266 {
              tunnel: [1.0 ("Value") -1.0 ("Value") 0.0 ("Value")] -> w265
              tunnel: [255.0 ("Value") 1.0 ("Value") 5.0 ("Value")] -> w264
              tunnel: [128.0 ("Value") 0.0 ("Value") 0.0 ("Value")] -> w263
              tunnel: [64.0 ("Value") 0.5 ("Value") 1.0 ("Value")] -> w262
              frame "PWM" {
              }
              frame "Motor", Default {
              }
              frame "Analog Out" {
              }
            }
            n140 = property on="Motor" class="Clust (strict)"("Visible"=TRUE) -> ()  [unwired: 2 in, 2 out]
            n141 = property on="Value" class="Slide (strict)"("Value"=w263, "Scale.Minimum"=w265, "Scale.Maximum"=w264, "Scale.Increment"=w262) -> ()  [unwired: 2 in, 2 out]
            n142 = property on="On/Off" class="Bool (strict)"("Visible"=w267) -> ()  [unwired: 2 in, 2 out]
            n143 = property on="Test Slider" class="Slide (strict)"("Visible"=w267) -> ()  [unwired: 2 in, 2 out]
            n144 = property on="Test Ring" class="Ring (strict)"("Visible"=w267) -> ()  [unwired: 2 in, 2 out]
            n145 = property on="Rev/Fwd" class="Clust (strict)"("Visible"=w267) -> ()  [unwired: 2 in, 2 out]
          }
          frame "Servo" {
            w283 = FALSE ("Visible")
            n146 = call <vilib>:"NT Read Number.vi"("Name"=w285) -> ("Numeric"=w284:dbl)  [unwired: 9 in, 1 out]
            n147 = property on="Test Slider" class="Slide (strict)"("Visible"=TRUE, "Scale.Maximum"=170.0 ("Scale.Range:Maximum")) -> ()  [unwired: 2 in, 2 out]
            n148 = local write "Test Slider"(w284) -> ()
            n149 = property on="Motor" class="Clust (strict)"("Visible"=w283) -> ()  [unwired: 2 in, 2 out]
            n150 = property on="Rev/Fwd" class="Clust (strict)"("Visible"=w283) -> ()  [unwired: 2 in, 2 out]
            n151 = property on="On/Off" class="Bool (strict)"("Visible"=w283) -> ()  [unwired: 2 in, 2 out]
            n152 = property on="Test Ring" class="Ring (strict)"("Visible"=w283) -> ()  [unwired: 2 in, 2 out]
          }
          frame "Relay", "Solenoid" {
            w286 = FALSE ("Visible")
            n153 = property on="Motor" class="Clust (strict)"("Visible"=w286) -> ()  [unwired: 2 in, 2 out]
            n154 = property on="Test Slider" class="Slide (strict)"("Visible"=w286) -> ()  [unwired: 2 in, 2 out]
            n155 = Search and Replace String(input string=w287, search string="/Value  **", replace string="/Direction") -> (result string=w293:string)  [unwired: 5 in, 3 out]
            n156 = property on="Test Ring" class="Ring (strict)"("Visible"=w286) -> ()  [unwired: 2 in, 2 out]
            n157 = call <vilib>:"NT Read String.vi"("Name"=w293) -> ("String"=w291:string)  [unwired: 9 in, 1 out]
            n158 = Equal?(x="Both directions", y=w291) -> (x = y?=w289:bool)
            n159 = Not(x=w289) -> (.not. x?=w290:bool)
            n160 = property on="Rev/Fwd" class="Clust (strict)"("Visible"=w289) -> ()  [unwired: 2 in, 2 out]
            n161 = property on="On/Off" class="Bool (strict)"("Visible"=w290, "Caption.Text"=w288) -> ()  [unwired: 2 in, 2 out]
          }
          frame "Compressor", "Digital Out" {
            w296 = FALSE ("Visible")
            # "Get direction and finish"
            n162 = property on="Motor" class="Clust (strict)"("Visible"=w296) -> ()  [unwired: 2 in, 2 out]
            n163 = property on="Test Slider" class="Slide (strict)"("Visible"=w296) -> ()  [unwired: 2 in, 2 out]
            n164 = property on="Test Ring" class="Ring (strict)"("Visible"=w296) -> ()  [unwired: 2 in, 2 out]
            n165 = property on="On/Off" class="Bool (strict)"("Visible"=TRUE, "Caption.Text"=w297) -> ()  [unwired: 2 in, 2 out]
            n166 = property on="Rev/Fwd" class="Clust (strict)"("Visible"=FALSE) -> ()  [unwired: 2 in, 2 out]
          }
          frame "Camera" {
            n167 = call <vilib>:"Get Last Path Segment.vi"("String in"=w304) -> ("String out"=w305:string)  [unwired: 10 in]
            n168 = property on="On/Off" class="Bool (strict)"("Visible"=FALSE) -> ()  [unwired: 2 in, 2 out]
            n169 = property on="Motor" class="Clust (strict)"("Visible"=FALSE) -> ()  [unwired: 2 in, 2 out]
            n170 = property on="Rev/Fwd" class="Clust (strict)"("Visible"=FALSE) -> ()  [unwired: 2 in, 2 out]
            n171 = case shown="\"White Balance  **\"" w305 {
              tunnel: w304 -> [w311 w320 w329 w338 w347 _ w353]
              tunnel: w303 -> [w309 w317 w326 w335 w344 _ _]
              frame "Size  **" {
                n172 = Index Array(array=w309) -> (element=w308:cluster{string[]})  [unwired: 1 in]
                n173 = call <vilib>:"NT Read String.vi"("Name"=w311) -> ("String"=w310:string)  [unwired: 9 in, 1 out]
                n174 = Unbundle(w308) -> (w306:string[])
                n175 = Match First String(2:w306, 3:w310) -> (0:w307:i32)  [unwired: 1 out]
                n176 = property on="Test Ring" class="Ring (strict)"("Value"=w307, "Strings []"=w306) -> ()  [unwired: 2 in, 2 out]
                n177 = property on="Test Ring" class="Ring (strict)"("Visible"=TRUE) -> ()  [unwired: 2 in, 2 out]
                n178 = property on="Test Slider" class="Slide (strict)"("Visible"=FALSE) -> ()  [unwired: 2 in, 2 out]
              }
              frame "White Balance  **" {
                n179 = Index Array(array=w317, index=1) -> (element=w318:cluster{string[]})
                n180 = call <vilib>:"NT Read String.vi"("Name"=w320) -> ("String"=w319:string)  [unwired: 9 in, 1 out]
                n181 = Unbundle(w318) -> (w315:string[])
                n182 = Match First String(2:w315, 3:w319) -> (0:w314:i32)  [unwired: 1 out]
                n183 = property on="Test Ring" class="Ring (strict)"("Value"=w314, "Strings []"=w315) -> ()  [unwired: 2 in, 2 out]
                n184 = property on="Test Ring" class="Ring (strict)"("Visible"=TRUE) -> ()  [unwired: 2 in, 2 out]
                n185 = property on="Test Slider" class="Slide (strict)"("Visible"=FALSE) -> ()  [unwired: 2 in, 2 out]
              }
              frame "Exposure  **" {
                n186 = Index Array(array=w326, index=2) -> (element=w327:cluster{string[]})
                n187 = call <vilib>:"NT Read String.vi"("Name"=w329) -> ("String"=w328:string)  [unwired: 9 in, 1 out]
                n188 = Unbundle(w327) -> (w323:string[])
                n189 = Match First String(2:w323, 3:w328) -> (0:w324:i32)  [unwired: 1 out]
                n190 = property on="Test Ring" class="Ring (strict)"("Value"=w324, "Strings []"=w323) -> ()  [unwired: 2 in, 2 out]
                n191 = property on="Test Ring" class="Ring (strict)"("Visible"=TRUE) -> ()  [unwired: 2 in, 2 out]
                n192 = property on="Test Slider" class="Slide (strict)"("Visible"=FALSE) -> ()  [unwired: 2 in, 2 out]
              }
              frame "Exposure Priority  **" {
                n193 = Index Array(array=w335, index=3) -> (element=w336:cluster{string[]})
                n194 = call <vilib>:"NT Read String.vi"("Name"=w338) -> ("String"=w337:string)  [unwired: 9 in, 1 out]
                n195 = Unbundle(w336) -> (w332:string[])
                n196 = Match First String(2:w332, 3:w337) -> (0:w333:i32)  [unwired: 1 out]
                n197 = property on="Test Ring" class="Ring (strict)"("Value"=w333, "Strings []"=w332) -> ()  [unwired: 2 in, 2 out]
                n198 = property on="Test Ring" class="Ring (strict)"("Visible"=TRUE) -> ()  [unwired: 2 in, 2 out]
                n199 = property on="Test Slider" class="Slide (strict)"("Visible"=FALSE) -> ()  [unwired: 2 in, 2 out]
              }
              frame "Color Enable  **" {
                n200 = Index Array(array=w344, index=4) -> (element=w345:cluster{string[]})
                n201 = call <vilib>:"NT Read String.vi"("Name"=w347) -> ("String"=w346:string)  [unwired: 9 in, 1 out]
                n202 = Unbundle(w345) -> (w341:string[])
                n203 = Match First String(2:w341, 3:w346) -> (0:w342:i32)  [unwired: 1 out]
                n204 = property on="Test Ring" class="Ring (strict)"("Value"=w342, "Strings []"=w341) -> ()  [unwired: 2 in, 2 out]
                n205 = property on="Test Ring" class="Ring (strict)"("Visible"=TRUE) -> ()  [unwired: 2 in, 2 out]
                n206 = property on="Test Slider" class="Slide (strict)"("Visible"=FALSE) -> ()  [unwired: 2 in, 2 out]
              }
              frame Default {
                n207 = property on="Test Ring" class="Ring (strict)"("Visible"=FALSE) -> ()  [unwired: 2 in, 2 out]
                n208 = property on="Test Slider" class="Slide (strict)"("Visible"=FALSE) -> ()  [unwired: 2 in, 2 out]
              }
              frame "Brightness  **", "Color Level  **", "Compression  **", "FPS  **", "Sharpness  **" {
                n209 = call <vilib>:"NT Read Number.vi"("Name"=w353) -> ("Numeric"=w352:dbl)  [unwired: 9 in, 1 out]
                n210 = local write "Test Slider"(w352) -> ()
                n211 = property on="Test Slider" class="Slide (strict)"("Visible"=TRUE, "Scale.Maximum"=100.0 ("Scale.Range:Maximum")) -> ()  [unwired: 2 in, 2 out]
                n212 = property on="Test Ring" class="Ring (strict)"("Visible"=FALSE) -> ()  [unwired: 2 in, 2 out]
              }
            }
          }
        }
        n213 = property on="Progress" class="Clust (strict)"("Visible"=FALSE) -> ()  [unwired: 2 in, 2 out]
      }
      event "Test Name": Mouse Enter {
        # "Populate the ring with the list of tests"
        n214 = event-data() -> ()  [unwired: 1 in, 1 out]
        n215 = call <vilib>:"NT Read String Array.vi"("Name"="/TestMode/TestList") -> ("String Array"=w361:string[])  [unwired: 9 in, 1 out]
        n216 = Build Array (concatenate)("Select the test to run...", w361) -> (w360:string[])
        n217 = property on="Test Name" class="Ring (strict)"("Strings []"=w360) -> ()  [unwired: 2 in, 2 out]
      }
      event "Test Name": Value Change {
        w363 = FALSE ("Visible")
        # "Tell the robot the test name to run"
        n218 = event-data() -> ("NewVal"=w367:u16)  [unwired: 1 in]
        n219 = property on="Test Name" class="Ring (strict)"() -> ("Strings []"=w368:string[])  [unwired: 2 in, 2 out]
        n220 = local write "Progress"(T6 {"Test Progress"=0, "Test Progress Text"=""} ("Progress")) -> ()
        n221 = Index Array(array=w368, index=w367) -> (element=w366:string)
        n222 = call <vilib>:"NT Write String.vi"("String"=w366, "Name"="/TestMode/TestName") -> ()  [unwired: 9 in, 1 out]
        n223 = property on="Progress" class="Clust (strict)"("Visible"=TRUE) -> ()  [unwired: 2 in, 2 out]
        n224 = property on="Motor" class="Clust (strict)"("Visible"=w363) -> ()  [unwired: 2 in, 2 out]
        n225 = property on="Test Slider" class="Slide (strict)"("Visible"=w363) -> ()  [unwired: 2 in, 2 out]
        n226 = property on="On/Off" class="Bool (strict)"("Visible"=w363) -> ()  [unwired: 2 in, 2 out]
        n227 = property on="Rev/Fwd" class="Clust (strict)"("Visible"=w363) -> ()  [unwired: 2 in, 2 out]
        n228 = property on="Test Ring" class="Ring (strict)"("Visible"=w363) -> ()  [unwired: 2 in, 2 out]
      }
      event "Select Auto": Mouse Enter {
        # "Populate the combo box with the list of autonomous options"
        n229 = event-data() -> ()  [unwired: 1 in, 1 out]
        n230 = call <vilib>:"NT Read String Array.vi"("Name"="Auto List") -> ("String Array"=w370:string[])  [unwired: 9 in, 1 out]
        n231 = property on="Select Auto" class="CmbBox"("Strings[]"=w370) -> ()  [unwired: 2 in, 2 out]
      }
      event "Select Auto": Value Change {
        # "User modified the Auto Selection. Write to NT variable so robot knows."
        n232 = event-data() -> ("NewVal"=w373:string)  [unwired: 1 in]
        n233 = call <vilib>:"NT Write String.vi"("String"=w373, "Name"="Auto Selector") -> ()  [unwired: 9 in, 1 out]
      }
      event "Command Selection": Value Change {
        # "Get the params and show in table"
        n234 = event-data() -> ("NewVal"=w379:i32)  [unwired: 1 in]
        n235 = property on="Command Selection" class="MCListbox (strict)"() -> ("ItemNames"=w377:string[][])  [unwired: 2 in, 2 out]
        n236 = call <vilib>:"WPI_DashboardUpdate Command Params.vi"("NewVal"=w379, "Commands"=w377, "Param Tbl"=w378) -> ()  [unwired: 8 in, 1 out]
      }
      event "Execute Command": Value Change {
        # "Started one, Unique ID holds\nresponse"
        n237 = event-data() -> ()  [unwired: 1 in, 1 out]
        n238 = property on="Command Selection" class="MCListbox (strict)"() -> ("ItemNames"=w390:string[][])  [unwired: 2 in, 2 out]
        n239 = Index Array(array=w390, index (row)="Command Selection", index (col)=0) -> (element=w388:string)
        n240 = call <vilib>:"Invoke Commands.vi"("Command Params"="Command Params", "Function Name"=w388) -> ("Params"=w384:u8, "Started"=w383:bool)  [unwired: 7 in, 1 out]
        n241 = Array Subset(array="Command Params", length (row)=w384) -> (w385:string[][])  [unwired: 3 in]
        n242 = Select(t="Executing" ("Cmd Status"), s=w383, f="" ("Cmd Status")) -> (s? t:f=→"Cmd Status":string)
      }
      event "Command Selection": Double Click {
        n243 = event-data() -> ("Row"=w398:i32)  [unwired: 1 in]
        n244 = property on="Command Selection" class="MCListbox (strict)"() -> ("ItemNames"=w401:string[][])  [unwired: 2 in, 2 out]
        n245 = local read "Command Params"() -> (w397:string[][])
        n246 = Index Array(array=w401, index (row)=w398, index (col)=0) -> (element=w399:string)
        n247 = call <vilib>:"Invoke Commands.vi"("Command Params"=w397, "Function Name"=w399) -> ("Params"=w396:u8, "Started"=w391:bool)  [unwired: 7 in, 1 out]
        n248 = Array Subset(array=w397, length (row)=w396) -> (w395:string[][])  [unwired: 3 in]
        n249 = Select(t="Executing" ("Cmd Status"), s=w391, f="" ("Cmd Status")) -> (s? t:f=w392:string)
        n250 = local write "Cmd Status"(w392) -> ()
      }
      event "CheckList": Double Click {
        # "Shift clears all"
        # "Update symbols on the listbox"
        n251 = event-data() -> ("PlatMods.Shift"=w403:bool, "Row"=w405:i32)  [unwired: 1 in]
        n252 = case shown="True" w403 {
          tunnel: w405 -> [w409 _]
          tunnel: 1 -> [w408 _]
          frame False {
            n253 = property on="CheckList" class="LstBox (strict)"() -> ("Item Symbols"=w407:i32[])  [unwired: 2 in, 2 out]
            n254 = Replace Array Subset(array=w407, new element=w408, index=w409) -> (w406:i32[])
            n255 = property on="CheckList" class="LstBox (strict)"("Item Symbols"=w406) -> ()  [unwired: 2 in, 2 out]
          }
          frame True {
            w410 = 0 ("Top Row")
            n256 = property on="CheckList" class="LstBox (strict)"() -> ("Number of Rows"=w412:u32)  [unwired: 2 in, 2 out]
            n257 = Initialize Array(0, w412) -> (w411:i32[])
            n258 = property on="CheckList" class="LstBox (strict)"("Top Row"=w410, "Value"=w410, "Item Symbols"=w411) -> ()  [unwired: 2 in, 2 out]
          }
        }
      }
      event "CheckList": Key Down {
        # "Update symbols on the listbox\nLeft and right keys check and uncheck"
        n259 = event-data() -> ("VKey"=w416:T19)  [unwired: 1 in]
        n260 = case shown="\"Left\", \"Right\"" w416 {
          selector: w416 -> [w421 _]
          tunnel: eventvkey."Left" ("VKey") -> [w419 _]
          frame "Left", "Right" {
            n261 = Equal?(x=w419, y=w421) -> (x = y?=w420:bool)
            n262 = Select(t=0, s=w420, f=1) -> (s? t:f=w422:i32)
            n263 = property on="CheckList" class="LstBox (strict)"() -> ("Item Symbols"=w425:i32[])  [unwired: 2 in, 2 out]
            n264 = Replace Array Subset(array=w425, new element=w422, index="CheckList") -> (w424:i32[])
            n265 = property on="CheckList" class="LstBox (strict)"("Item Symbols"=w424) -> ()  [unwired: 2 in, 2 out]
          }
          frame Default {
          }
        }
      }
      event "Motor.Enable": Value Change {
        # "When the test mode otor enable helper is set, update that\ntree row item's value"
        n266 = event-data() -> ("NewVal"=w431:bool)  [unwired: 1 in]
        n267 = Unbundle("Motor") -> ("Value"=w430:dbl)  [unwired: 1 out]
        n268 = Select(t=w430, s=w431, f=0.0) -> (s? t:f=w428:dbl)
        n269 = call <vilib>:"NT Write Number.vi"("Numeric"=w428, "Name"=w427) -> ()  [unwired: 9 in, 1 out]
      }
      event "Test Slider": Value Change {
        # "When the test mode slider helper is set, update that\ntree row item's value"
        n270 = event-data() -> ("NewVal"=w434:dbl)  [unwired: 1 in]
        n271 = call <vilib>:"NT Write Number.vi"("Numeric"=w434, "Name"=w435) -> ()  [unwired: 9 in, 1 out]
      }
      event "On/Off": Value Change {
        # "When the test mode on/off helper value is set, update that\ntree row item's value"
        n272 = event-data() -> ("NewVal"=w439:bool)  [unwired: 1 in]
        n273 = Boolean To (0,1)(Boolean=w439) -> (0, 1=w438:i16)
        n274 = call <vilib>:"NT Write Number.vi"("Numeric"=w438, "Name"=w437) -> ()  [unwired: 9 in, 1 out]
      }
      event "Rev/Fwd": Value Change {
        # "When the test mode helper value for relays is set, update that\ntree row item's value"
        n275 = event-data() -> ("NewVal.Forward"=w447:bool, "NewVal.Reverse"=w446:bool)  [unwired: 1 in]
        n276 = Boolean To (0,1)(Boolean=w447) -> (0, 1=w443:i16)
        n277 = Boolean To (0,1)(Boolean=w446) -> (0, 1=w445:i16)
        n278 = Negate(x=w445) -> (-x=w444:i16)
        n279 = Add(x=w443, y=w444) -> (x+y=w442:i16)
        n280 = call <vilib>:"NT Write Number.vi"("Numeric"=w442, "Name"=w441) -> ()  [unwired: 9 in, 1 out]
      }
      event "Test Ring": Value Change {
        # "When a test mode helper value is selected from the ring,\nset the tree item's variable to the string value"
        n281 = event-data() -> ("NewVal"=w451:u16)  [unwired: 1 in]
        n282 = property on="Test Ring" class="Ring (strict)"() -> ("Strings []"=w452:string[])  [unwired: 2 in, 2 out]
        n283 = Index Array(array=w452, index=w451) -> (element=w450:string)
        n284 = call <vilib>:"NT Write String.vi"("String"=w450, "Name"=w449) -> ()  [unwired: 9 in, 1 out]
      }
      event "Rec Mode": Value Change {
        # "Update globals for recording mode and path to read log from.\nClear when logging and let NetworkTables set path for vision to\nuse."
        n285 = event-data() -> ("NewVal"=w463:enum32{"Stop", "Record", "Playback"})  [unwired: 1 in]
        n286 = global write "WPI_DashboardLogging Global.vi" "Logging Filename"(path "") -> ()
        n287 = global write "WPI_DashboardLogging Global.vi" "Recording"(w463) -> ()
        n288 = case shown="\"Playback\"" w463 {
          tunnel: w462 -> [_ w465 w474]
          tunnel: [_ _ w473] -> w460
          tunnel: [_ _ w472] -> _
          tunnel: w458 -> [_ _ w470]
          tunnel: cluster{i32, i32} {-250, 170} -> [_ _ w469]
          tunnel: [_ _ T20 {"Image Size"=TRUE, "Image Type"=TRUE, "Pixel Value"=TRUE, "ROI Information"=TRUE, "Zoom Factor"=FALSE} ("Image Information Shown:All Elements")] -> w456
          tunnel: [_ _ TRUE ("Zoom Factor")] -> w455
          tunnel: w454 -> [_ _ w466]
          frame Default {
          }
          frame "Stop", "Record" {
            # "Place Window too"
            n289 = invoke class="VI" method="FP.Close"(reference=w465) -> (reference out=w464:refnum<vi>)  [unwired: 2 in, 2 out]
            n290 = invoke class="VI" method="Abort VI"(reference=w464) -> ()  [unwired: 2 in, 3 out]
          }
          frame "Playback" {
            n291 = call "Open Playback Panel.vi"("Offset"=w469, "DB VI Ref"=w470, "Playback in"=w474) -> ("Playback out"=w471:refnum<vi>)  [unwired: 8 in]
            n292 = register-events(w471, w466) -> (reference out=w473:refnum<event-registration>, error out=w472:errorcluster)  [unwired: 2 in]
          }
        }
        n293 = property on="Camera Image" class="ImageControl"("Image Information Shown"=w456, "Image Information Visible"=w455) -> ()  [unwired: 2 in, 2 out]
        n294 = call <vilib>:"WPI_DashboardNT Log FieldName Cache.vi"("Operation"=enum16{"Lookup/Add", "Index", "Clear"}."Clear") -> ()  [unwired: 8 in, 3 out]
      }
      event Panel Close {
        w476 = enum32{"Stop", "Record", "Playback"}."Stop" ("Rec Mode")
        # "Playback window has been closed, abort"
        n295 = event-data() -> ()  [unwired: 1 in, 4 out]
        n296 = local write "Rec Mode"(w476) -> ()
        n297 = global write "WPI_DashboardLogging Global.vi" "Recording"(w476) -> ()
      }
      event Panel Close {
        # "Abort playback window and ourself"
        n298 = event-data() -> ()  [unwired: 1 in, 4 out]
        n299 = invoke class="VI" method="FP.Close"(reference=w480) -> (reference out=w479:refnum<vi>)  [unwired: 2 in, 2 out]
        n300 = invoke class="VI" method="Abort VI"(reference=w479) -> (error out=w478:errorcluster)  [unwired: 2 in, 2 out]
        n301 = invoke class="VI" method="Abort VI"(error in=w478) -> ()  [unwired: 2 in, 3 out]
      }
      event User Event {
        n302 = event-data() -> ("IDs"=w487:cluster{"RPC field ID":u16, "Unique ID":u16}, "String"=w486:string)  [unwired: 1 in]
        n303 = Bundle("IDs"=w487, "String"=w486) -> (w485:T8)  [unwired: 1 in]
        n304 = call <vilib>:"Retrieve RPC Response.vi"("RPC Response"=w485) -> ("Output"=w483:string[][])  [unwired: 10 in]
        n305 = Build Array (concatenate)(w481, w483) -> (w482:string[][])
        n306 = local write "Command Params"(w482) -> ()
        n307 = local write "Cmd Status"("" ("Cmd Status")) -> ()
      }
      event "Tree": Double Click {
        n308 = event-data() -> ("PlatMods"=w491:T23, "Tag"=w490:string)  [unwired: 1 in]
        n309 = Unbundle(w491) -> ("Shift"=w489:bool)  [unwired: 4 out]
        n310 = Not(x=w489) -> (.not. x?=w488:bool)
        n311 = call <vilib>:"NT Update Persistence.vi"("Persistence"=w488, "Name"=w490) -> ()  [unwired: 9 in, 1 out]
      }
    }
  }
  n312 = while {
    tunnel: w76 -> [w494]
    i -> [w497]
    stop <- FALSE stop-if-true
    n313 = Wait (ms)(milliseconds to wait=u32 100) -> ()  [unwired: 1 out]
    n314 = case shown="\"Playback\"" "Rec Mode" {
      tunnel: w497 -> [_ _ w512]
      tunnel: [u32 2829099 ("Base Color") u32 11141120 ("Target Color") w501] -> w493
      frame "Stop", Default {
        # "Reset the color, extra updates don't cost much"
      }
      frame "Record" {
      }
      frame "Playback" {
        # "Playback"
        n315 = Quotient & Remainder(x=w512, y=u32 50 ("milliseconds to wait")) -> (x-y*floor(x/y)=w508:u32)  [unwired: 1 out]
        n316 = Divide(x=w508, y=u32 50 ("milliseconds to wait")) -> (x/y=w505:dbl)
        n317 = Multiply(x=6.283185307179586, y=w505) -> (x*y=w510:dbl)
        n318 = Sine(x=w510) -> (sin(x)=w509:dbl)
        n319 = Absolute Value(x=w509) -> (abs(x)=w502:dbl)
        n320 = call "Interpolate RGB Color.vi"("Proportion"=w502, "Target Color"=u32 30976, "Base Color"=u32 2829099) -> ("Result Color"=w501:u32)  [unwired: 8 in]
      }
    }
    n321 = property class="Pane"(reference=w494, "PaneColor"=w493) -> ()  [unwired: 1 in, 2 out]
  }
  n322 = local write "Dashboard Tab"(T2."Drive" ("Dashboard Tab")) -> ()
  n323 = property on="On/Off" class="Bool (strict)"("Visible"=w47) -> ()  [unwired: 2 in, 2 out]
  n324 = property on="Motor" class="Clust (strict)"("Visible"=w47) -> ()  [unwired: 2 in, 2 out]
  n325 = property on="Progress" class="Clust (strict)"("Visible"=w47) -> ()  [unwired: 2 in, 2 out]
  n326 = property on="Test Ring" class="Ring (strict)"("Visible"=w47) -> ()  [unwired: 2 in, 2 out]
  n327 = property on="Rev/Fwd" class="Clust (strict)"("Visible"=w47) -> ()  [unwired: 2 in, 2 out]
  n328 = call-poly <vilib>:"NT Read Value.vi"("Name"="ZAcc") -> ("Numeric"=→"Z Acceleration":dbl)  [unwired: 9 in, 1 out]
  n329 = call-poly <vilib>:"NT Read Value.vi"("Name"="YAcc") -> ("Numeric"=→"Y Acceleration":dbl)  [unwired: 9 in, 1 out]
  n330 = call-poly <vilib>:"NT Read Value.vi"("Name"="XAcc") -> ("Numeric"=→"X Acceleration":dbl)  [unwired: 9 in, 1 out]
  n331 = while {
    tunnel: u16 1741 ("timeout ms (25000)") -> [w514]
    stop <- FALSE stop-if-true
    n332 = TCP Create Listener(10:w514) -> (0:w513:errorcluster, 3:w515:refnum<k5>)  [unwired: 4 in, 1 out]
    n333 = case shown="No Error" w513 {
      selector: w513 -> [w517 _]
      tunnel: w515 -> [w518 _]
      frame No Error {
        n334 = while {
          tunnel: w518 -> [w521]
          tunnel: w517 -> [w520]
          stop <- FALSE stop-if-true
          n335 = TCP Wait On Listener(8:w520, 11:w521) -> (0:w522:errorcluster, 4:w523:refnum<k5>)  [unwired: 2 in, 3 out]
          n336 = local write "TCP"(w523) -> ()
          n337 = case shown="No Error" w522 {
            frame No Error {
            }
            frame Error {
              n338 = Wait (ms)(milliseconds to wait=u32 1000) -> ()  [unwired: 1 out]
            }
          }
        }
      }
      frame Error {
        n339 = Wait (ms)(milliseconds to wait=u32 1000) -> ()  [unwired: 1 out]
      }
    }
  }
  n340 = local write "Command Selection"(u16 0 ("milliseconds to wait")) -> ()
  n341 = local write "Command Params"(string[][] [] ("Command Params")) -> ()
  n342 = global write "WPI_DashboardLogging Global.vi" "Recording"(w70) -> ()
  n343 = local write "Rec Mode"(w70) -> ()
  n344 = call <vilib>:"NT Write String.vi"("String"="Select Auto", "Name"="Auto Selector") -> ()  [unwired: 9 in, 1 out]
  n345 = while {
    stop <- "Calculate Angle" stop-if-true
    n346 = formula code="Angle=O/H;\nA=(sin(Angle));"("O"="Distance from \nthe lift to the wall", "H"="Distance from\n lift to corner", "Angle"=1.0 ("input variable")) -> ("A"=→"Angle":dbl)
  }
  n347 = call-poly <vilib>:"NT Read Value.vi"("Name"="Sonar") -> ("Numeric"=→"distance":dbl)  [unwired: 9 in, 1 out]
  n348 = call-poly <vilib>:"NT Write Value.vi"("Numeric"="Smooth", "Name"="Smooth") -> ()  [unwired: 9 in, 1 out]
  n349 = call-poly <vilib>:"NT Write Value.vi"("Numeric"="Scaling factor (V/in)", "Name"="Scaling") -> ()  [unwired: 9 in, 1 out]
